vi "Default Components Directory.vi"() -> (3 "Default Components Directory":path)   [LabVIEW 2019, in "DSF Core.lvlib" / "Framework.lvclass"]
uses:
  Classes/Framework/Framework.lvclass
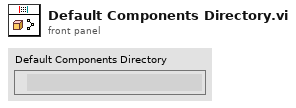
[diagram p1: front panel]
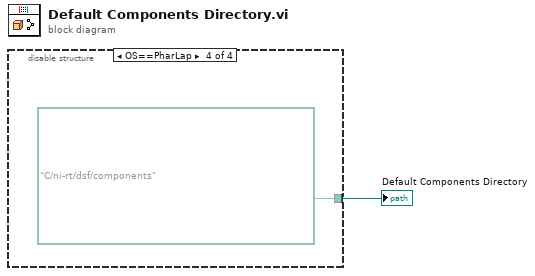
[diagram p0: block diagram]
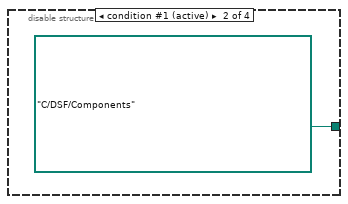
[diagram p3: hidden frame]
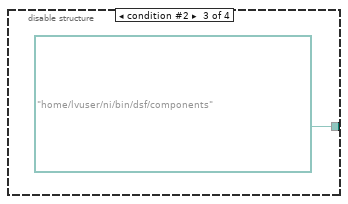
[diagram p4: hidden frame]
diagram:
  n1 = disable-structure shown="OS==PharLap" {
    disable-tunnel: [_ path "C:/DSF/Components" ("transceivers directory") path "/home/lvuser/ni/bin/dsf/components" ("transceivers directory") path "C:/ni-rt/dsf/components" ("transceivers directory")] -> w1
    frame condition #0 {
    }
    frame condition #1 (active) {
    }
    frame condition #2 {
    }
    frame condition #3 {
    }
  }
  "Default Components Directory" <- w1
